vi "Update Value Control.vi"(8 "error in (no error)":errorcluster, 11 "Camera Settings Dialog in":refnum<class "Camera Settings Dialog.lvclass">) -> (0 "error out":errorcluster, 3 "Camera Settings Dialog out":refnum<class "Camera Settings Dialog.lvclass">)   [LabVIEW 2020, in "Camera Settings Dialog UI.lvlib" / "Camera Settings Dialog.lvclass"]
uses:
  Camera Settings Dialog.lvclass
  Camera Settings Dialog.lvclass/Camera Settings Dialog.ctl
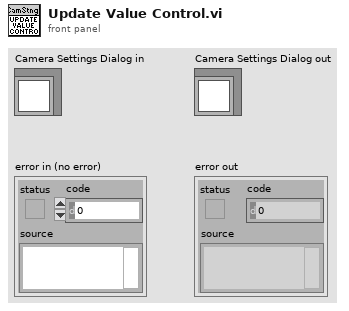
[diagram p1: front panel]
types:
  T1 = typedef "Camera Attribute Info.ctl" = cluster{"Attribute Type":string, "Readable":bool, "Writable":bool, "Attribute Name":string, "DisplayName":string, "Units":string, "Tooltip":string, "ValueString":string, "MaxDBL":dbl, "MaxI64":i64, "MaxString":string, "MaxU32":u32, "MinDBL":dbl, "MinI64":i64, "MinString":string, "MinU32":u32, "ValueBool":bool, "ValueDBL":dbl, "ValueI64 ":i64, "ValueString":string, "ValueU32":u32, "IncDBL":dbl, "IncU32":u32, "IncI64":i64, "EnumStrings":string[], "EnumValues":u32[]}
  T2 = cluster{"Tab Control":refnum<vi>, "U32 Value Control":refnum<vi>, "DBL Value Control":refnum<vi>, "String Value Control":refnum<vi>, "Enum Value Control":refnum<vi>, "Boolean Value Control":refnum<vi>, "Command Value Control":refnum<vi>}
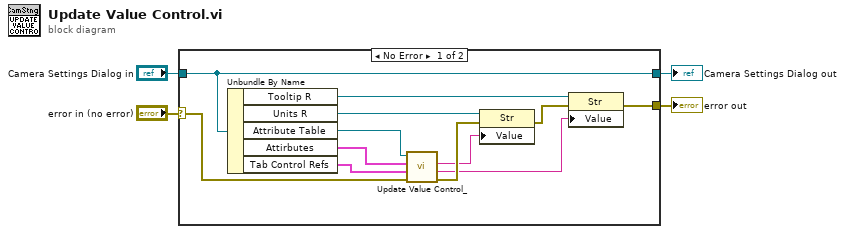
[diagram p0: block diagram]
diagram:
  n1 = case shown="No Error" "error in (no error)" {
    selector: "error in (no error)" -> [w11 w18]
    tunnel: [w5 w18] -> w3
    tunnel: [w15 w17] -> w1
    tunnel: "Camera Settings Dialog in" -> [w15 w17]
    frame No Error {
      n2 = Unbundle By Name(w15) -> ("Tooltip R"=w10:refnum<vi>, "Units R"=w8:refnum<vi>, "Attribute Table"=w12:refnum<vi>, "Attirbutes"=w13:T1[], "Tab Control Refs"=w14:T2)
      n3 = call "Update Value Control_.vi"("error in (no error)"=w11, "Tab Control Ref In"=w14, "Attirbutes"=w13, "Tree Control In"=w12) -> ("error out"=w16:errorcluster, "Tooltip"=w9:string, "Units"=w7:string)  [unwired: 5 in]
      n4 = property class="Str"(reference=w8, error in=w16, "Value"=w7) -> (error out=w6:errorcluster)  [unwired: 1 out]
      n5 = property class="Str"(reference=w10, error in=w6, "Value"=w9) -> (error out=w5:errorcluster)  [unwired: 1 out]
    }
    frame Error {
    }
  }
  "error out" <- w3
  "Camera Settings Dialog out" <- w1
